vi "Register Nested.vi"(8 "error in (no error)":errorcluster, 9 "Module ID":string, 10 "MessageQ":refnum<class "MessageQ.lvclass">, 11 "Module in":refnum<class "Module.lvclass">) -> (0 "error out":errorcluster, 3 "Module out":refnum<class "Module.lvclass">)   [LabVIEW 2020, in "Volatus.lvlib" / "Module.lvclass"]
uses:
  Module.lvclass
  MessageQ/MessageQ.lvclass
  Module.lvclass/Module.ctl
  Module Status Update.ctl
  State.ctl
  Volatus.lvlib
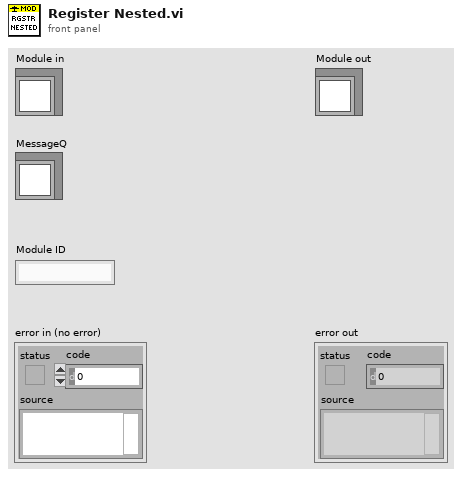
[diagram p1: front panel]
types:
  T1 = typedef "Volatus.lvlib/Module Status Update.ctl" = cluster{"MessageQ":refnum<class "MessageQ.lvclass">, "State":T2, "Hierarchy":string[], "Forwarded":bool}
  T2 = typedef "Volatus.lvlib/Module.lvclass/State.ctl" = enum16{"Unknown", "Launched", "Starting", "Running", "Stopping", "Stopped", "Error - Starting", "Error - Run", "Error - Stopping"}
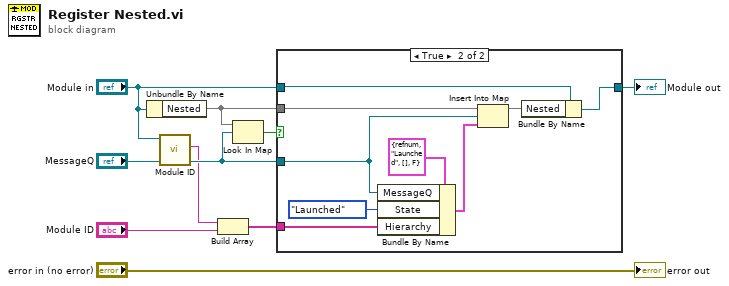
[diagram p0: block diagram]
diagram:
  n1 = Unbundle By Name("Module in") -> ("Nested"=w7:map{refnum<class "MessageQ.lvclass">, T1})
  n2 = call-dynamic "Module ID.vi"("Module in"="Module in") -> ("Module ID"=w3:string)  [unwired: 10 in]
  n3 = Build Array(w3, "Module ID") -> (w1:string[])
  n4 = Look In Map(map=w7, key="MessageQ") -> (key not found?=w5:bool)  [unwired: 1 in, 1 out]
  n5 = case shown="True" w5 {
    tunnel: w7 -> [_ w17]
    tunnel: "MessageQ" -> [_ w12]
    tunnel: "Module in" -> [w10 w19]
    tunnel: [w10 w18] -> w8
    tunnel: w1 -> [_ w11]
    frame False {
    }
    frame True {
      n6 = Bundle By Name(cluster=T1 {"MessageQ"=refnum, "State"=enum."Launched", "Hierarchy"=[], "Forwarded"=FALSE} ("value"), "MessageQ"=w12, "State"=State."Launched", "Hierarchy"=w11) -> (w14:T1)
      n7 = Insert Into Map(map in=w17, key=w12, value=w14) -> (map out=w16:map{refnum<class "MessageQ.lvclass">, T1})  [unwired: 2 out]
      n8 = Bundle By Name(cluster=w19, "Nested"=w16) -> (w18:refnum<class "Module.lvclass">)
    }
  }
  "Module out" <- w8
  "error out" <- "error in (no error)"
